vi "helper_GetRegistrationInfo-MultisitePinMapA.vi"(10 "Pin Map ID":string) -> (2 "Reservation Request Info":T3(array[cluster]))   [LabVIEW 2020]
uses:
  Runtime/MeasurementLink Session Management Client/RPC Messages/ni_measurementlink_sessionmanagement_v1_ReserveSessionsRequest.ctl
  Runtime/MeasurementLink Session Management Client/RPC Messages/ni_measurementlink_PinMapContext.ctl
  Runtime/MeasurementLink Session Management Client/MeasurementLink Session Management Client.lvlib
panel:
  out "Reservation Request Data (both DCPower & Scope)":T1[](array[typedef])
  out "Reservation Request Data (Scope only)":T1[](array[typedef])
  out "Reservation Request Data (DCPower only)":T1[](array[typedef])
  # "This helper builds session management registration info (and associated 'expected' session / instrument info) for the test pinmap dubbed \"MultisitePinMapA\""
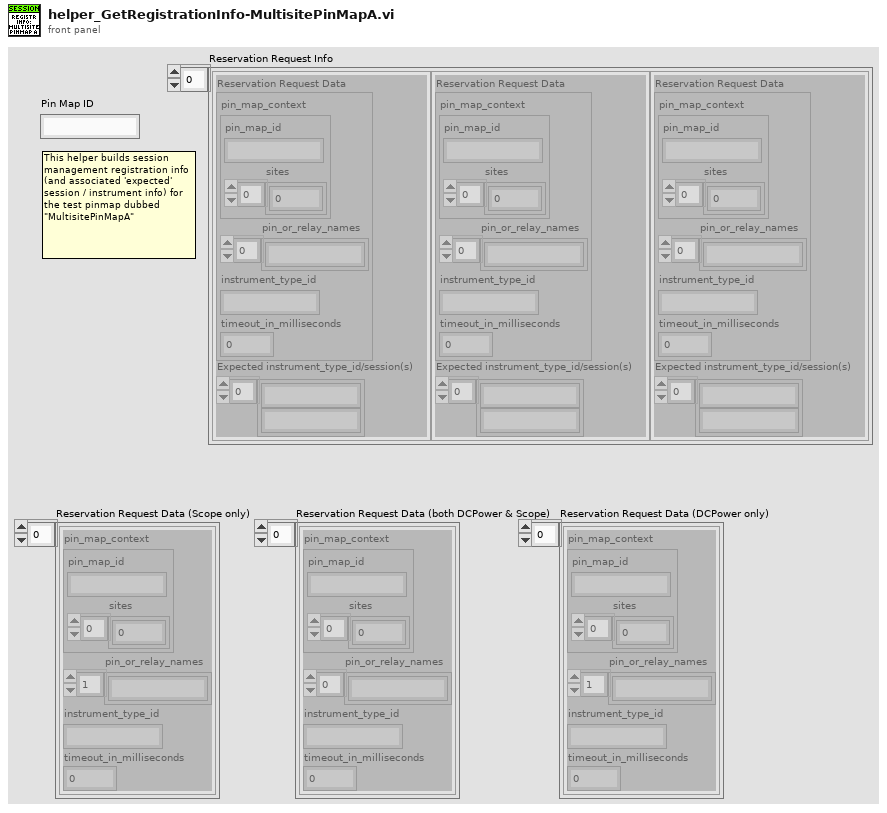
[diagram p1: front panel]
types:
  T1 = typedef "MeasurementLink Session Management Client.lvlib/ni_measurementlink_sessionmanagement_v1_ReserveSessionsRequest.ctl" = cluster{"pin_map_context":T2, "pin_or_relay_names":string[], "instrument_type_id":string, "timeout_in_milliseconds":i32}
  T2 = typedef "MeasurementLink Session Management Client.lvlib/ni_measurementlink_PinMapContext.ctl" = cluster{"pin_map_id":string, "sites":i32[]}
  T3 = cluster{"Reservation Request Data":T1, "Expected instrument_type_id/session(s)":string[]}[]
  T4 = cluster{"Reservation Request Data":T1, "Expected instrument_type_id/session(s)":string[]}
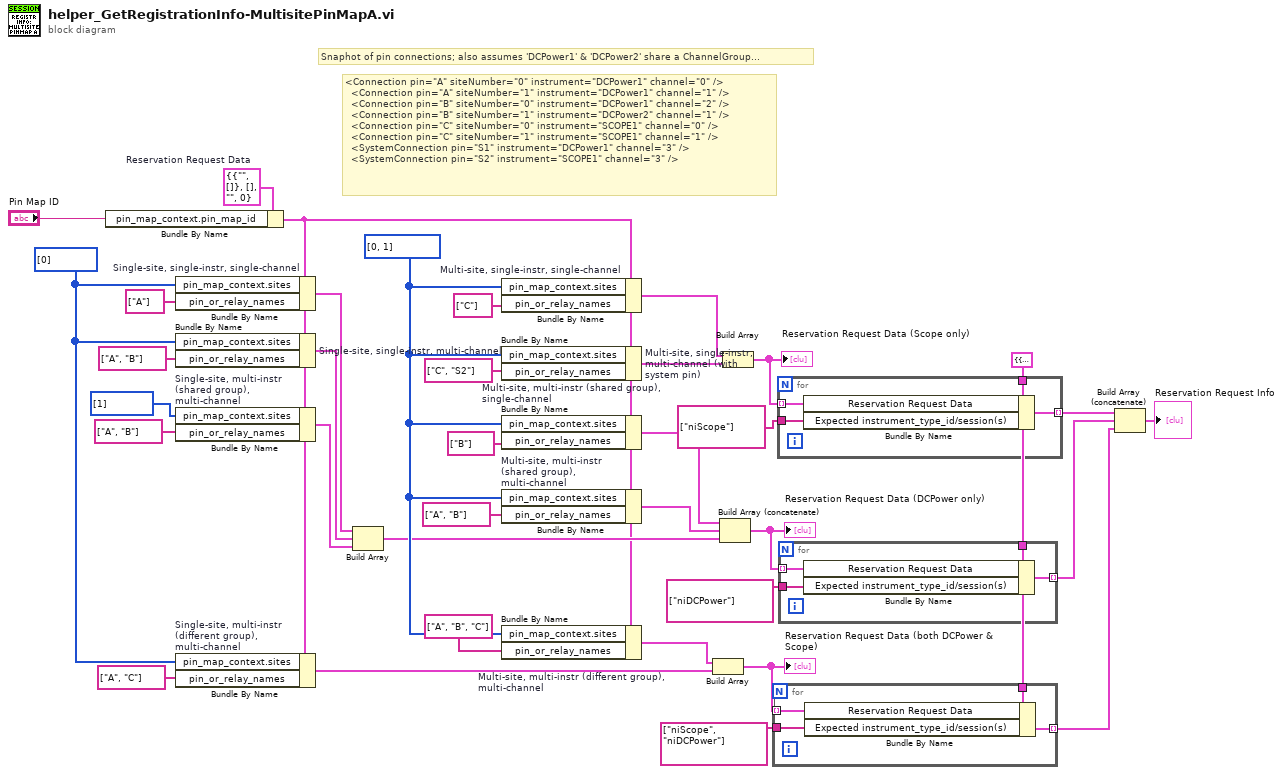
[diagram p0: block diagram]
diagram:
  w8 = T4 {"Reservation Request Data"={"pin_map_context"={"pin_map_id"="", "sites"=[]}, "pin_or_relay_names"=[], "instrument_type_id"="", "timeout_in_milliseconds"=0}, "Expected instrument_type_id/session(s)"=[]}
  w22 = i32[] [0, 1] ("pin_map_context.sites")
  w35 = T1 {"pin_map_context"={"pin_map_id"="", "sites"=[]}, "pin_or_relay_names"=[], "instrument_type_id"="", "timeout_in_milliseconds"=0}  # Reservation Request Data
  w25 = i32[] [0] ("pin_map_context.sites")
  # "Snaphot of pin connections; also assumes 'DCPower1' & 'DCPower2' share a ChannelGroup..."
  # "<Connection pin=\"A\" siteNumber=\"0\" instrument=\"DCPower1\" channel=\"0\" />\n\t\t<Connection pin=\"A\" siteNumber=\"1\" instrument=\"DCPower1\" channel=\"1\" />\n\t\t<Connection pin=\"B\" siteNumber=\"0\" instrument=\"DCPower1\" channel=\"2\" />\n\t\t<Connection pin=\"B\" siteNumber=\"1\" instrument=\"DCPower2\" channel=\"1\" />\n\t\t<Connection pin=\"C\" siteNumber=\"0\" instrument=\"SCOPE1\" channel=\"0\" />\n\t\t<Connection pin=\"C\" siteNumber=\"1\" instrument=\"SCOPE1\" channel=\"1\" />\n\t\t<SystemConnection pin=\"S1\" instrument=\"DCPower1\" channel=\"3\" />\n\t\t<SystemConnection pin=\"S2\" instrument=\"SCOPE1\" channel=\"3\" />"
  n1 = Bundle By Name(cluster=w35, "pin_map_context.pin_map_id"="Pin Map ID") -> (w14:T1)
  n2 = Bundle By Name "Single-site, single-instr, single-channel"(cluster=w14, "pin_map_context.sites"=w25, "pin_or_relay_names"=string[] ["A"]) -> (w27:T1)
  n3 = Bundle By Name "Single-site, single-instr, multi-channel"(cluster=w14, "pin_map_context.sites"=w25, "pin_or_relay_names"=string[] ["A", "B"]) -> (w26:T1)
  n4 = Bundle By Name "Single-site, multi-instr (shared group), multi-channel"(cluster=w14, "pin_map_context.sites"=i32[] [1], "pin_or_relay_names"=string[] ["A", "B"]) -> (w21:T1)
  n5 = Bundle By Name "Single-site, multi-instr (different group), multi-channel"(cluster=w14, "pin_map_context.sites"=w25, "pin_or_relay_names"=string[] ["A", "C"]) -> (w18:T1)
  n6 = Build Array(w27, w26, w21) -> (w17:T1[])
  n7 = Bundle By Name "Multi-site, single-instr, single-channel"(cluster=w14, "pin_map_context.sites"=w22, "pin_or_relay_names"=string[] ["C"]) -> (w13:T1)
  n8 = Bundle By Name "Multi-site, single-instr, multi-channel (with system pin)"(cluster=w14, "pin_map_context.sites"=w22, "pin_or_relay_names"=string[] ["C", "S2"]) -> (w12:T1)
  n9 = Bundle By Name "Multi-site, multi-instr (shared group), single-channel"(cluster=w14, "pin_map_context.sites"=w22, "pin_or_relay_names"=string[] ["B"]) -> (w15:T1)
  n10 = Bundle By Name "Multi-site, multi-instr (shared group), multi-channel"(cluster=w14, "pin_map_context.sites"=w22, "pin_or_relay_names"=string[] ["A", "B"]) -> (w16:T1)
  n11 = Bundle By Name "Multi-site, multi-instr (different group), multi-channel"(cluster=w14, "pin_map_context.sites"=w22, "pin_or_relay_names"=string[] ["A", "B", "C"]) -> (w19:T1)
  n12 = Build Array(w19, w18) -> (w9:T1[])
  "Reservation Request Data (both DCPower & Scope)" <- w9
  n13 = Build Array (concatenate)(w15, w16, w17) -> (w10:T1[])
  "Reservation Request Data (DCPower only)" <- w10
  n14 = Build Array(w13, w12) -> (w11:T1[])
  "Reservation Request Data (Scope only)" <- w11
  n15 = for {
    tunnel: w9 -> [w39] mode=indexing
    tunnel: w8 -> [w40]
    tunnel: [w38] -> w5 mode=indexing
    tunnel: string[] ["niScope", "niDCPower"] -> [w37]
    n16 = Bundle By Name(cluster=w40, "Reservation Request Data"=w39, "Expected instrument_type_id/session(s)"=w37) -> (w38:T4)
  }
  n17 = for {
    tunnel: w11 -> [w43] mode=indexing
    tunnel: w8 -> [w44]
    tunnel: [w42] -> w7 mode=indexing
    tunnel: string[] ["niScope"] -> [w41]
    n18 = Bundle By Name(cluster=w44, "Reservation Request Data"=w43, "Expected instrument_type_id/session(s)"=w41) -> (w42:T4)
  }
  n19 = for {
    tunnel: w10 -> [w47] mode=indexing
    tunnel: w8 -> [w48]
    tunnel: [w46] -> w6 mode=indexing
    tunnel: string[] ["niDCPower"] -> [w45]
    n20 = Bundle By Name(cluster=w48, "Reservation Request Data"=w47, "Expected instrument_type_id/session(s)"=w45) -> (w46:T4)
  }
  n21 = Build Array (concatenate)(w7, w6, w5) -> (→"Reservation Request Info":T3)
